vi "SetImageDisplayPallete.vi"(8 "Error In":errorcluster, 11 "Value":T1) -> (0 "Error Out":errorcluster, 3 "Palette:Palette Type":u32)   [LabVIEW 2015]
uses:
  Controls/UI_Process_Type.ctl
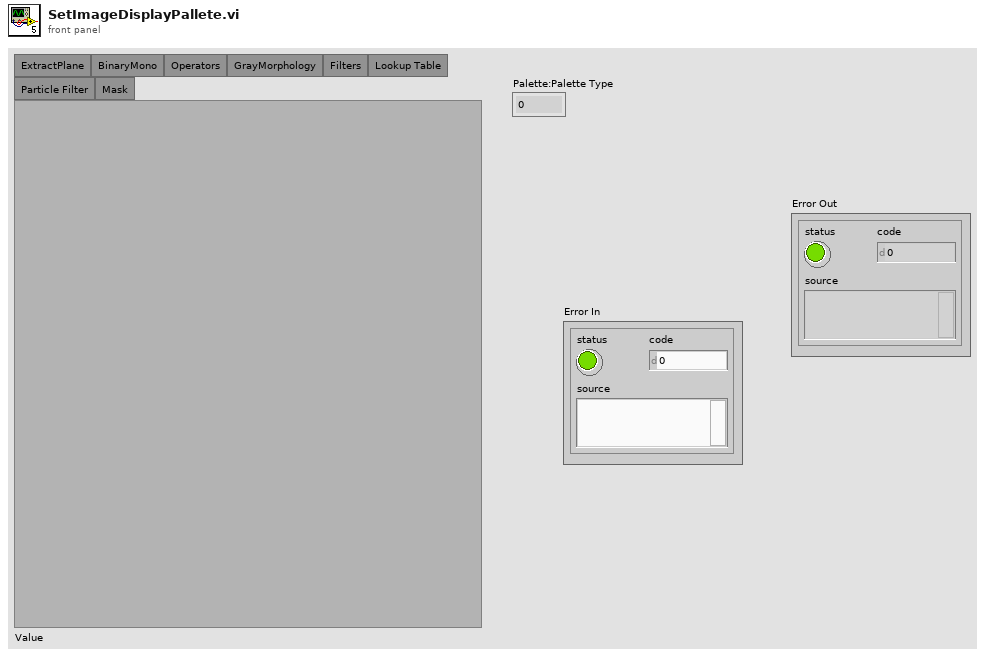
[diagram p1: front panel]
types:
  T1 = typedef "UI_Process_Type.ctl" = enum32{"None", "ExtractPlane", "BinaryMono", "Operators", "GrayMorphology", "Filters", "Lookup Table", "Particle Filter", "Mask"}
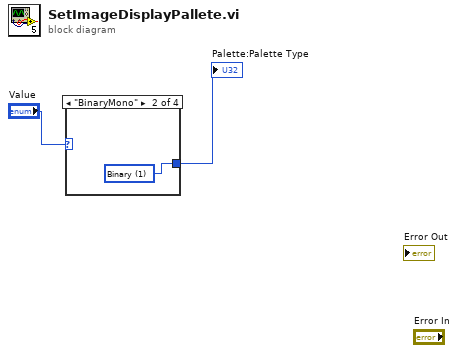
[diagram p0: block diagram]
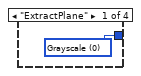
[diagram p2: hidden frame]
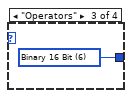
[diagram p3: hidden frame]
diagram:
  n1 = case shown="\"BinaryMono\"" "Value" {
    tunnel: [w3 w4 w5 _] -> w1
    frame "ExtractPlane" {
      w3 = u32 0 items=["Grayscale", "Binary", "Gradient", "Rainbow", "Temperature", "User Defined", "Binary 16 Bit", "Gradient 16 Bit", "Rainbow 16 Bit", "Temperature 16 Bit", "User Defined 16 Bit"] ("Palette:Palette Type")
    }
    frame "BinaryMono" {
      w4 = u32 1 items=["Grayscale", "Binary", "Gradient", "Rainbow", "Temperature", "User Defined", "Binary 16 Bit", "Gradient 16 Bit", "Rainbow 16 Bit", "Temperature 16 Bit", "User Defined 16 Bit"] ("Palette:Palette Type")
    }
    frame "Operators" {
      w5 = u32 6 items=["Grayscale", "Binary", "Gradient", "Rainbow", "Temperature", "User Defined", "Binary 16 Bit", "Gradient 16 Bit", "Rainbow 16 Bit", "Temperature 16 Bit", "User Defined 16 Bit"] ("Palette:Palette Type")
    }
    frame "None", Default {
    }
  }
  "Palette:Palette Type" <- w1
